vi "OPC Check.vi"() -> ()   [LabVIEW 2020]
uses:
  Controls/OP20B_DataCluster.ctl
panel:
  out "Array":string[](array[string])
  out "Array 4":bool[](array[boolean])
  out "[CIRCLIP_POS_MIN]":dbl
  out "[CIRCLIP_POS]":dbl
  out "[CIRCLIP_POS_MAX]":dbl
  out "[CIRCLIP_POS_STATUS]":dbl
  out "[PREACTUATOR_TRAVEL_MIN]":dbl
  out "[PREACTUATOR_TRAVEL]":dbl
  out "[PREACTUATOR_TRAVEL_MAX]":dbl
  out "[PREACTUATOR_TRAVEL_STATUS]":dbl
  out "[CT]":dbl
  out "OP20B_004_PREACTUATION":T1
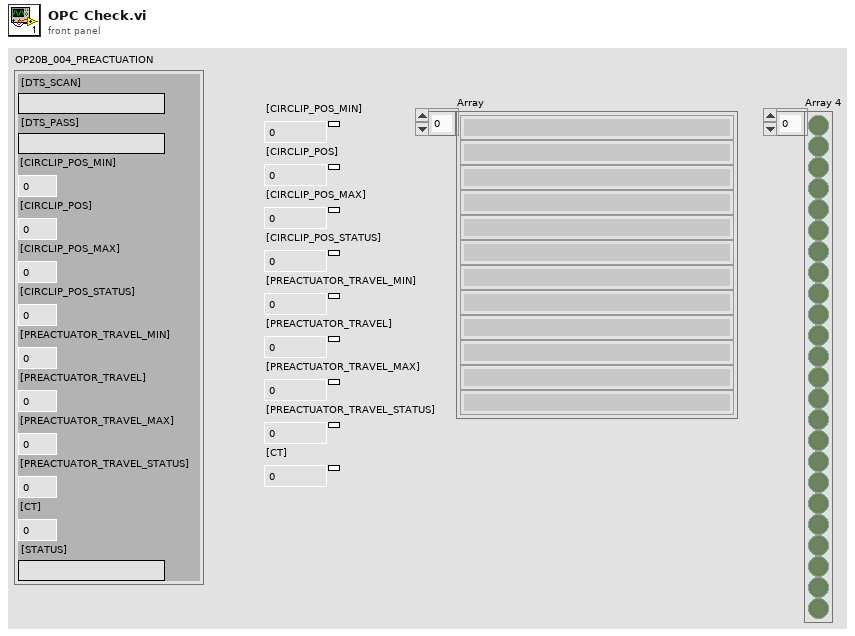
[diagram p1: front panel]
types:
  T1 = typedef "OP20B_DataCluster.ctl" = cluster{"[DTS_SCAN]":string, "[DTS_PASS]":string, "[CIRCLIP_POS_MIN]":dbl, "[CIRCLIP_POS]":dbl, "[CIRCLIP_POS_MAX]":dbl, "[CIRCLIP_POS_STATUS]":dbl, "[PREACTUATOR_TRAVEL_MIN]":dbl, "[PREACTUATOR_TRAVEL]":dbl, "[PREACTUATOR_TRAVEL_MAX]":dbl, "[PREACTUATOR_TRAVEL_STATUS]":dbl, "[CT]":dbl, "[STATUS]":string}
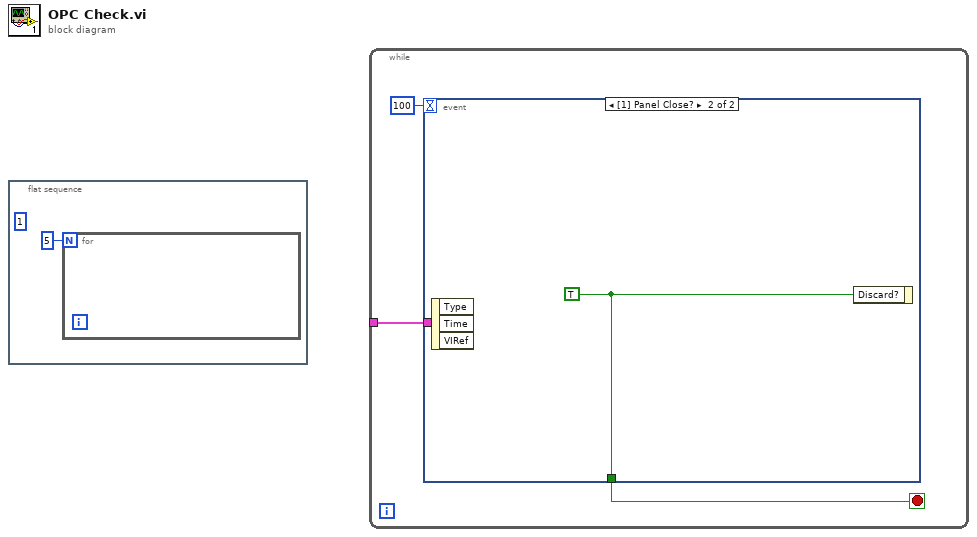
[diagram p0: block diagram]
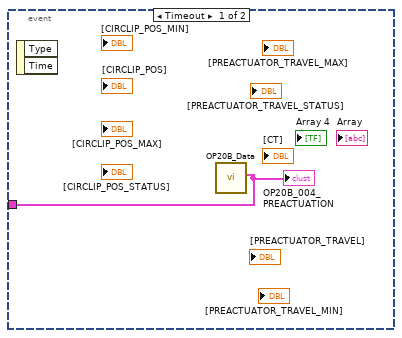
[diagram p2: hidden frame]
diagram:
  n1 = flat-sequence {
    frame #0 {
      (unwired) 1
      n2 = for {
        N: 5 -> [_]
      }
    }
  }
  n3 = while {
    tunnel: [w2] -> _
    stop <- w4 stop-if-true
    n4 = event shown="[1] Panel Close?" {
      selector: _ -> [_ _]
      dyn-events: _ -> [_ _]
      timeout: 100 -> [_ _]
      tunnel: [_ w6] -> w4
      tunnel: [w5 _] -> w2
      event Timeout {
        n5 = event-data() -> ()  [unwired: 1 in, 2 out]
        n6 = call "OP20B_Data.vi"() -> ("OP20B_004_PREACTUATION"=w5:T1)  [unwired: 9 in]
        "OP20B_004_PREACTUATION" <- w5
      }
      event Panel Close? {
        w6 = TRUE ("Discard?")
        n7 = event-data() -> ()  [unwired: 1 in, 3 out]
        n8 = event-data("Discard?"=w6) -> ()  [unwired: 1 in, 1 out]
      }
    }
  }
